vi "Generate Certificate.vi"() -> ()   [LabVIEW 2013]
doc: "Generates a self-signed CA server certificate and private key file."
uses:
  <vilib>/Utility/sysdir.llb/System Directory Type.ctl
panel:
  out "resulting string":string
  out "standard output":string
  out "standard error":string
  in  "2-Letter Country Code":string
  in  "Certificate File (.crt)":path
  in  "Private Key File Path (.key)":path
  in  "Common Name":string
  in  "Validity (days)":i32=3560
  in  "Alternate Names":string[](array[string])
  in  "Path to openssl":path=path "C:/Program Files (x86)/National Instruments/Shared/nissl/openssl.exe"
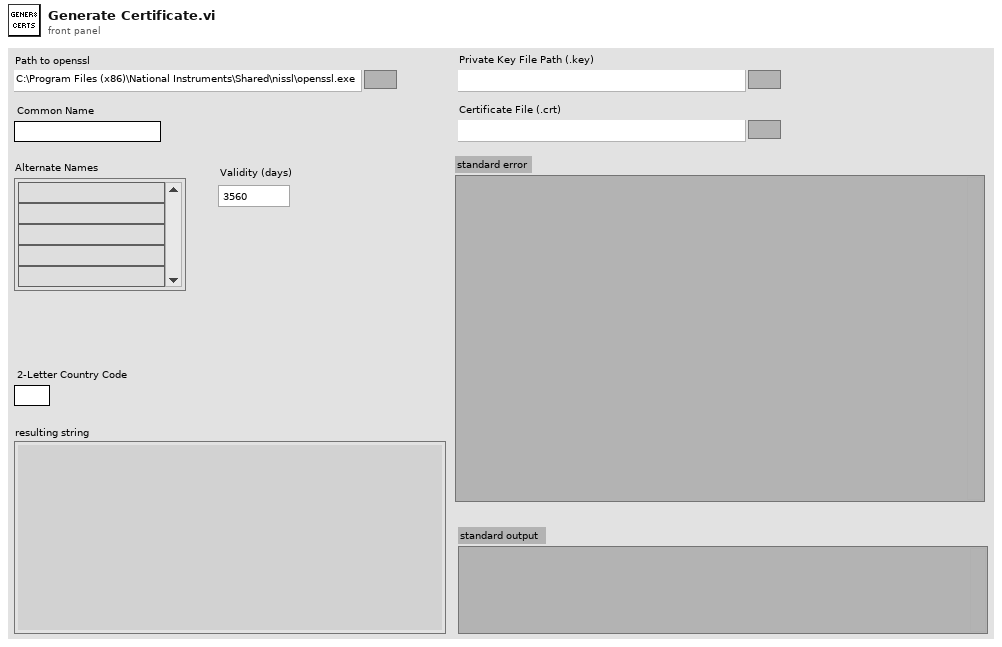
[diagram p1: front panel]
types:
  T1 = typedef "System Directory Type.ctl" = i32
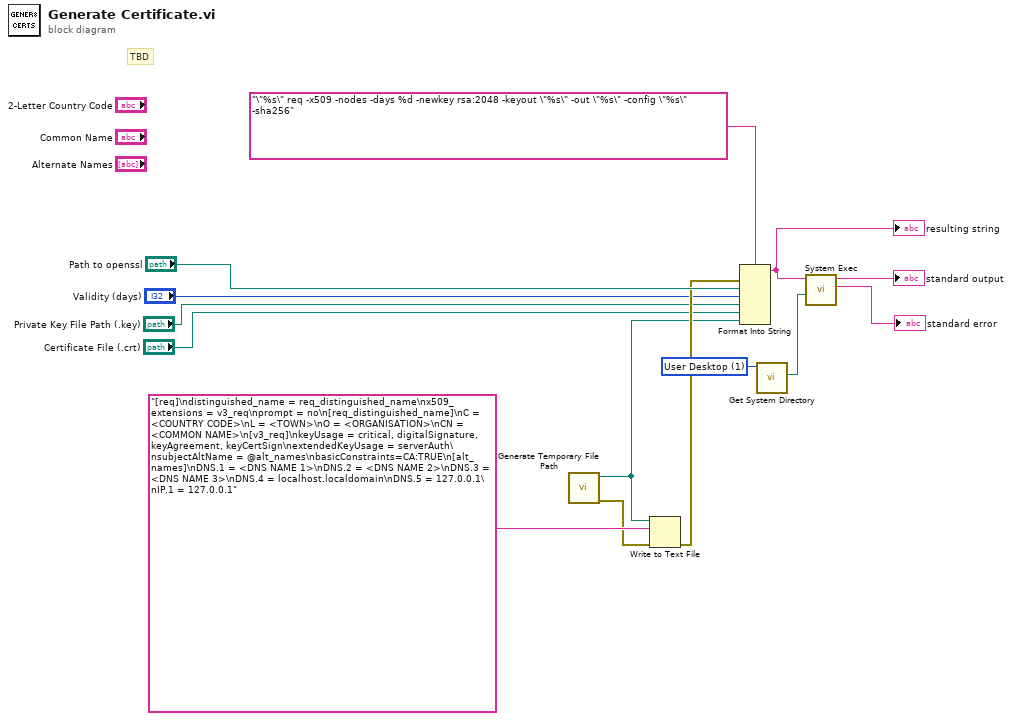
[diagram p0: block diagram]
diagram:
  w2 = T1 1 items=["User Home"=0, "User Desktop"=1, "User Documents"=2, "User Application Data"=3, "User Preferences"=4, "User Temporary"=5, "Public Documents"=6, "Public Application Data"=7, "Public Preferences"=8, "Public Cache"=13, "System Core Libraries"=9, "System Installed Libraries"=10, "Application Files"=11, "Boot Volume Root"=12] ("system directory type")
  # "TBD"
  n1 = call <vilib>:"Generate Temporary File Path.vi"() -> ("error out"=w9:errorcluster, "Unique Temporary File Path"=w6:path)  [unwired: 10 in]
  n2 = Write to Text File(file (use dialog)=w6, text="[req]\ndistinguished_name = req_distinguished_name\nx509_extensions = v3_req\nprompt = no\n[req_distinguished_name]\nC = <COUNTRY CODE>\nL = <TOWN>\nO = <ORGANISATION>\nCN = <COMMON NAME>\n[v3_req]\nkeyUsage = critical, digitalSignature, keyAgreement, keyCertSign\nextendedKeyUsage = serverAuth\nsubjectAltName = @alt_names\nbasicConstraints=CA:TRUE\n[alt_names]\nDNS.1 = <DNS NAME 1>\nDNS.2 = <DNS NAME 2>\nDNS.3 = <DNS NAME 3>\nDNS.4 = localhost.localdomain\nDNS.5 = 127.0.0.1\nIP.1 = 127.0.0.1", error in=w9) -> (error out=w8:errorcluster)  [unwired: 1 in, 2 out]
  n3 = Format Into String(format string="\"%s\" req -x509 -nodes -days %d -newkey rsa:2048 -keyout \"%s\" -out \"%s\" -config \"%s\" -sha256", error in=w8, "Path to openssl", "Validity (days)", "Private Key File Path (.key)", "Certificate File (.crt)", w6) -> (resulting string=w7:string)  [unwired: 1 in, 1 out]
  "resulting string" <- w7
  n4 = call <vilib>:"Get System Directory.vi"("system directory type"=w2) -> ("system directory"=w1:path)  [unwired: 10 in]
  n5 = call <vilib>:"System Exec.vi"("working directory"=w1, "command line"=w7) -> ("standard error"=→"standard error":string, "standard output"=→"standard output":string)  [unwired: 6 in, 2 out]
